vi "Get Or Create Typedef.vi"(8 "error in (no error)":errorcluster, 9 "Create cluster inside Typedef?":bool, 10 "Name":string, 11 "Library in":refnum<vi>) -> (0 "error out":errorcluster, 1 "Cluster ref out":refnum<vi>, 2 "VI ref out":refnum<vi>, 3 "Library out":refnum<vi>, 5 "Path":path)   [LabVIEW 2025, in "gRPC Template Creation Utility.lvlib"]
uses:
  gRPC Template Creation Utility.lvlib
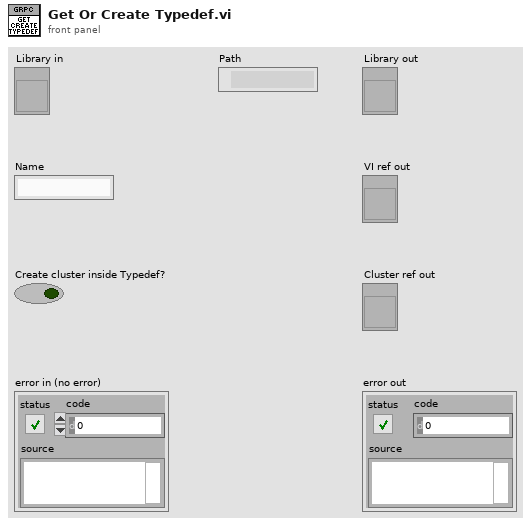
[diagram p1: front panel]
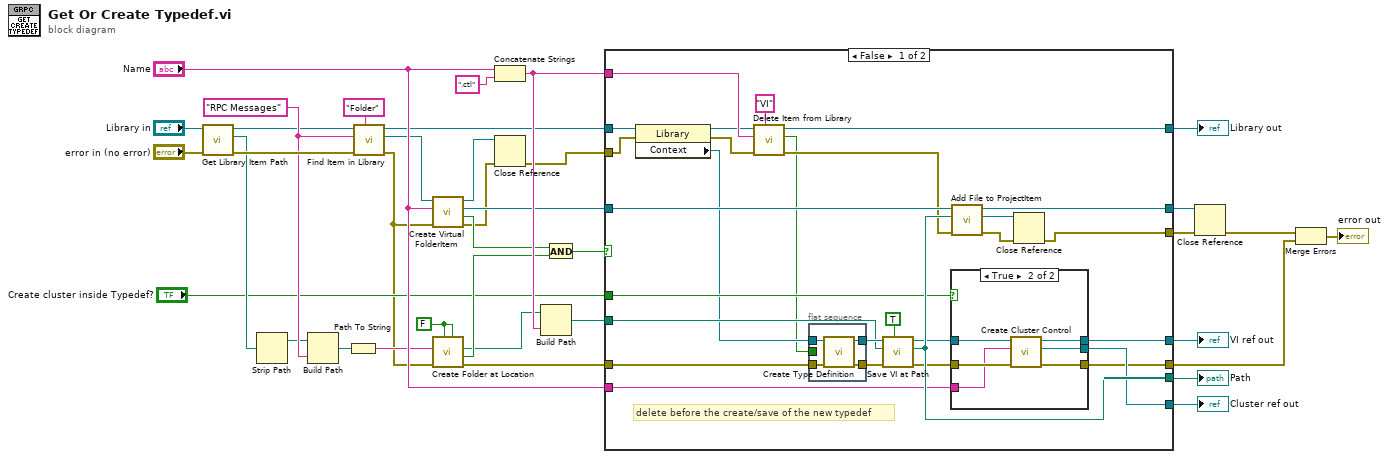
[diagram p0: block diagram]
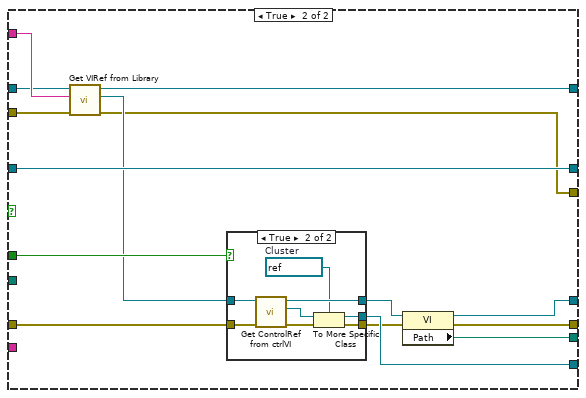
[diagram p3: hidden frame]
diagram:
  w22 = "RPC Messages" ("Item Name")
  w6 = FALSE ("Use Relative")
  n1 = call "Get Library Item Path.vi"("error in (no error)"="error in (no error)", "Library"="Library in") -> ("error out"=w23:errorcluster, "Path"=w16:path, "Library"=w21:refnum<vi>)  [unwired: 7 in]
  n2 = Strip Path(path=w16) -> (stripped path=w15:path)  [unwired: 1 out]
  n3 = Build Path(base path=w15, name or relative path=w22) -> (appended path=w36:path)
  n4 = Path To String(path=w36) -> (string=w13:string)
  n5 = call "Find Item in Library.vi"("Item Type"="Folder", "error in (no error)"=w23, "Item Name"=w22, "Library item in"=w21) -> ("error out"=w1:errorcluster, "Project Item (Library Item)"=w20:refnum<vi>, "Library item out"=w27:refnum<vi>)  [unwired: 4 in, 1 out]
  n6 = call "Create Virtual FolderItem.vi"("error in (no error)"=w1, "Folder Name"="Name", "ProjectItem in"=w20) -> ("error out"=w4:errorcluster, "Already exists?"=w30:bool, "FolderItem reference out"=w26:refnum<vi>, "ProjectItem out"=w3:refnum<vi>)  [unwired: 5 in]
  n7 = call "Create Folder at Location.vi"("Override existing (F)"=w6, "Use Relative (F)"=w6, "Error In"=w1, "Path"=w13) -> ("Error Out"=w14:errorcluster, "Already Exists ?"=w31:bool, "Full path out"=w12:path)  [unwired: 5 in]
  n8 = Concatenate Strings("Name", ".ctl" ("string")) -> (w34:string)
  n9 = Close Reference(reference=w3, error in (no error)=w4) -> (error out=w2:errorcluster)
  n10 = Build Path(base path=w12, name or relative path=w34) -> (appended path=w25:path)
  n11 = And(x=w30, y=w31) -> (x .and. y?=w32:bool)
  n12 = case shown="False" w32 {
    tunnel: w14 -> [w65 w80]
    tunnel: [w47 w90] -> w18
    tunnel: [w64 w83] -> w37
    tunnel: [w63 w78] -> w9
    tunnel: w25 -> [w61 _]
    tunnel: w26 -> [w59 w88]
    tunnel: w27 -> [w43 w87]
    tunnel: [w44 w92] -> w28
    tunnel: [w57 w88] -> w11
    tunnel: w34 -> [w52 w89]
    tunnel: [w58 w91] -> w29
    tunnel: w2 -> [w41 w81]
    tunnel: [w56 w79] -> w10
    tunnel: "Name" -> [w49 _]
    tunnel: "Create cluster inside Typedef?" -> [w48 w86]
    frame False {
      # "delete before the create/save of the new typedef"
      n13 = property class="Library"(reference=w43, error in=w41) -> (reference out=w42:refnum<vi>, error out=w40:errorcluster, "Context"=w39:refnum<vi>)
      n14 = call "Delete Item from Library.vi"("Item Type"="VI", "error in (no error)"=w40, "Item name"=w52, "Library"=w42) -> ("error out"=w51:errorcluster, "Deleted ?"=w38:bool, "Library"=w44:refnum<vi>)  [unwired: 5 in]
      n15 = flat-sequence {
        tunnel: w65 -> [w69]
        tunnel: [w68] -> w62
        tunnel: [w67] -> w60
        tunnel: w39 -> [w66]
        tunnel: w38 -> [_]
        frame #0 {
          n16 = call "Create Type Definition.vi"("error in (no error)"=w69, "application"=w66) -> ("error out"=w67:errorcluster, "TypeDef VI out"=w68:refnum<vi>)  [unwired: 8 in]
        }
      }
      n17 = call "Save VI at Path.vi"("Override Existing? (T)"=TRUE, "error in (no error)"=w60, "Path"=w61, "VI in"=w62) -> ("error out"=w55:errorcluster, "Path to saved File"=w58:path, "VI out"=w54:refnum<vi>)  [unwired: 5 in]
      n18 = case shown="True" w48 {
        tunnel: [_ w77] -> w64
        tunnel: [w71 w76] -> w63
        tunnel: w55 -> [w71 w75]
        tunnel: w54 -> [w70 w74]
        tunnel: w49 -> [_ w73]
        tunnel: [w70 w72] -> w47
        frame False {
        }
        frame True {
          n19 = call "Create Cluster Control.vi"("error in (no error)"=w75, "Cluster Label"=w73, "Owning vi in"=w74) -> ("error out"=w76:errorcluster, "Cluster ref out"=w77:refnum<vi>, "Owning vi out"=w72:refnum<vi>)  [unwired: 6 in]
        }
      }
      n20 = call "Add File to ProjectItem.vi"("error in (no error)"=w51, "File Path"=w58, "ProjectItem in"=w59) -> ("error out"=w45:errorcluster, "Added File ref"=w46:refnum<vi>, "ProjectItem out"=w57:refnum<vi>)  [unwired: 6 in]
      n21 = Close Reference(reference=w46, error in (no error)=w45) -> (error out=w56:errorcluster)
    }
    frame True {
      n22 = call "Get VIRef from Library.vi"("error in (no error)"=w81, "item name"=w89, "library in"=w87) -> ("error out"=w79:errorcluster, "vi"=w85:refnum<vi>, "library out"=w92:refnum<vi>)  [unwired: 5 in, 1 out]
      n23 = case shown="True" w86 {
        tunnel: w80 -> [w93 w102]
        tunnel: w85 -> [w94 w101]
        tunnel: [w94 w99] -> w84
        tunnel: [_ w96] -> w83
        tunnel: [w93 w95] -> w82
        frame False {
        }
        frame True {
          w98 = refnum<vi> refnum  # Cluster
          n24 = call "Get ControlRef from ctrlVI.vi"("error in (no error)"=w102, "VI ref in"=w101) -> ("error out"=w100:errorcluster, "Control ref out"=w97:refnum<vi>, "VI ref out"=w99:refnum<vi>)  [unwired: 7 in]
          n25 = To More Specific Class(target class=w98, reference=w97, error in=w100) -> (specific class reference=w96:refnum<vi>, error out=w95:errorcluster)
        }
      }
      n26 = property class="VI"(reference=w84, error in=w82) -> (reference out=w90:refnum<vi>, error out=w78:errorcluster, "Path"=w91:path)
    }
  }
  "Cluster ref out" <- w37
  "Path" <- w29
  "Library out" <- w28
  "VI ref out" <- w18
  n27 = Close Reference(reference=w11, error in (no error)=w10) -> (error out=w5:errorcluster)
  n28 = Merge Errors(w5, w9) -> (→"error out":errorcluster)
